vi "formatBackslashCodeSubVI.vi"(8 "error in (no error)":errorcluster, 11 "Endian":T1=enum."Little") -> (0 "error out":errorcluster, 3 "Values":string[](array[string]))   [LabVIEW 2019, in "Instrument Addon Unit Tests.lvclass"]
doc: "Generates an array of values for each data type for the following numeric to string configuratio:\nChannel Type: Type Cast\nEndian: [User defined]\nNumeric value: 1"
uses:
  Instrument Addon Unit Tests.lvclass
  Addon/Addon Shared/Types/Endian.ctl
  Addon/Addon Shared/Types/Type Cast Type.ctl
  Addon/Addon Shared/Types/Metadata Channel Type.ctl
  Addon/Addon Engine/Instrument Addon Engine.lvlib
  Addon/Addon Shared/Instrument Addon Shared.lvlib
panel:
  out "Value Read":string
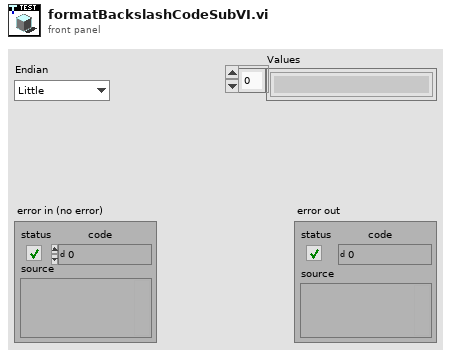
[diagram p1: front panel]
types:
  T1 = typedef "Instrument Addon Shared.lvlib/Endian.ctl" = enum16{"Native", "Little", "Big"}
  T2 = typedef "Instrument Addon Shared.lvlib/Metadata Channel Type.ctl" = enum16{"Enumerated List", "Format", "Type Cast"}
  T3 = typedef "Instrument Addon Shared.lvlib/Type Cast Type.ctl" = enum16{"DBL", "SGL", "U64", "U32", "U16", "U8", "I64", "I32", "I16", "I8"}
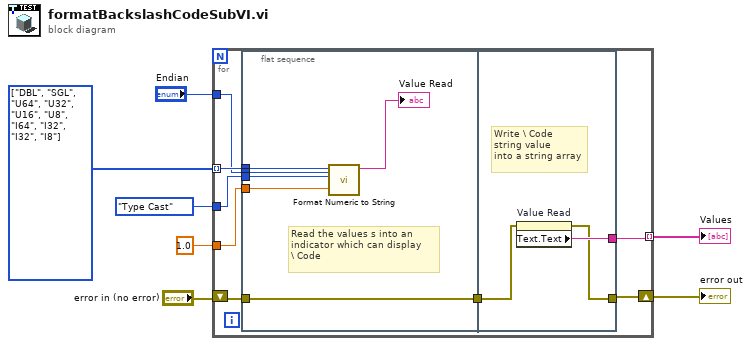
[diagram p0: block diagram]
diagram:
  w7 = T3[] [enum."DBL", enum."SGL", enum."U64", enum."U32", enum."U16", enum."U8", enum."I64", enum."I32", enum."I32", enum."I8"] items=["DBL", "SGL", "U64", "U32", "U16", "U8", "I64", "I32", "I16", "I8"]
  n1 = for {
    tunnel: w7 -> [w15] mode=indexing
    tunnel: "Endian" -> [w14]
    tunnel: Metadata_Channel_Type."Type Cast" ("Channel Type") -> [w13]
    tunnel: 1.0 ("Numeric") -> [w12]
    tunnel: [w11] -> w3 mode=indexing
    shift-right: [w8] -> w1
    shift-left: "error in (no error)" -> [w9]
    n2 = flat-sequence {
      tunnel: w15 -> [w21]
      tunnel: w14 -> [w20]
      tunnel: w13 -> [w19]
      tunnel: w12 -> [w18]
      tunnel: [w16] -> w10
      tunnel: w9 -> [w16]
      tunnel: [w24] -> w11
      tunnel: w10 -> [w23]
      tunnel: [w22] -> w8
      frame #0 {
        # "Read the values s into an\nindicator which can display \n\\ Code"
        n3 = call "Format Numeric to String.vi"("Numeric"=w18, "Endian"=w20, "Channel Type"=w19, "Type"=w21) -> ("Value"=→"Value Read":string)  [unwired: 7 in]
      }
      frame #1 {
        # "Write \\ Code\nstring value \ninto a string array"
        n4 = property on="Value Read" class="Str"(error in=w23) -> (error out=w22:errorcluster, "Text.Text"=w24:string)  [unwired: 1 in, 1 out]
      }
    }
  }
  "Values" <- w3
  "error out" <- w1
